vi "generate true.vi"() -> (3 "json string":string)   [LabVIEW 2013, in "json generator.lvlib"]
uses:
  json generator.lvlib
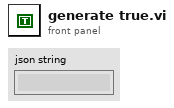
[diagram p1: front panel]
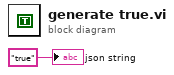
[diagram p0: block diagram]
diagram:
  "json string" <- "true" ("json string")
